vi "Load Variables.vi"(6 "Constants":refnum<class "Sequence Constants.lvclass">, 8 "error in (no error)":refnum<class "MultiErrors.lvclass">, 10 "Config Element":refnum<class "Config Element.lvclass">) -> (0 "error out":refnum<class "MultiErrors.lvclass">, 2 "Variables":map{string, T1}(c390))   [LabVIEW 2020, in "VolatusSeqConfig.lvlib" / "Sequence Config.lvclass"]
uses:
  Sequence Config.lvclass
  VolatusErrorUtilities/MultiErrors/MultiErrors.lvclass
  lv-cdm/CDM-Config/Config Element/Config Element.lvclass
  Variable.ctl
  VolatusErrorUtilities/MultiErrors/MultiErrors.lvclass/MultiErrors.ctl
  Sequence Config.lvclass/Sequence Config.ctl
  VolatusSeqConfig.lvlib
  Sequence Constants/Sequence Constants.lvclass
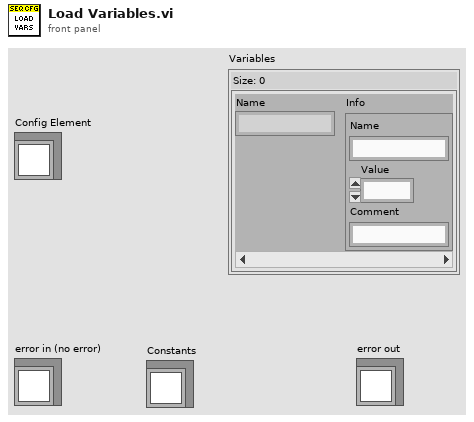
[diagram p1: front panel]
types:
  T1 = typedef "VolatusSeqConfig.lvlib/Variable.ctl" = cluster{"Name":string, "Value":dbl, "Comment":string}
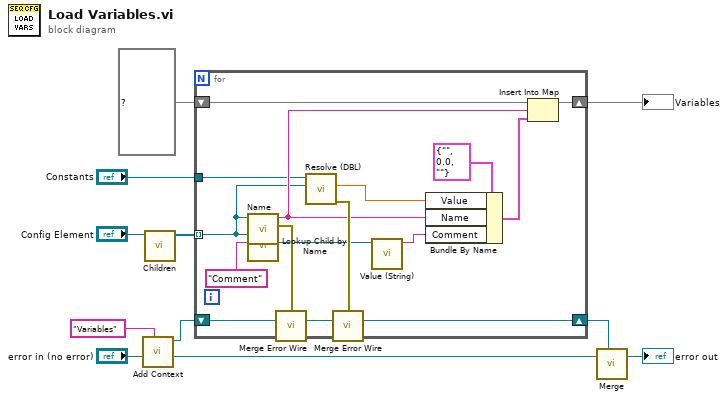
[diagram p0: block diagram]
diagram:
  n1 = call "Add Context.vi"("Context"="Variables", "MultiErrors in"="error in (no error)") -> ("Original Context"=w4:refnum<class "MultiErrors.lvclass">, "Added Context"=w3:refnum<class "MultiErrors.lvclass">)  [unwired: 8 in]
  n2 = call "Children.vi"("Config Element in"="Config Element") -> ("Elements"=w10:refnum<class "Config Element.lvclass">[])  [unwired: 9 in, 1 out]
  n3 = for {
    tunnel: w10 -> [w13] mode=indexing
    shift-right: [w23] -> w8
    shift-left: map{string, T1} {} ("Variables") -> [w24]
    shift-right: [w15] -> w6
    shift-left: w3 -> [w17]
    tunnel: "Constants" -> [w14]
    n4 = call "Name.vi"("Config Element in"=w13) -> ("error out"=w26:errorcluster, "Name"=w21:string)  [unwired: 9 in]
    n5 = call "Lookup Child by Name.vi"("Name"="Comment", "Config Element in"=w13) -> ("Child"=w19:refnum<class "Config Element.lvclass">)  [unwired: 6 in, 3 out]
    n6 = call "Merge Error Wire.vi"("error in (no error)"=w26, "MultiErrors in"=w17) -> ("MultiErrors out"=w16:refnum<class "MultiErrors.lvclass">)  [unwired: 13 in]
    n7 = call "Resolve (DBL).vi"("Element"=w13, "Sequence Constants in"=w14) -> ("error out"=w27:errorcluster, "DBL Value"=w12:dbl)  [unwired: 7 in, 1 out]
    n8 = call "Merge Error Wire.vi"("error in (no error)"=w27, "MultiErrors in"=w16) -> ("MultiErrors out"=w15:refnum<class "MultiErrors.lvclass">)  [unwired: 13 in]
    n9 = call "Value (String).vi"("Config Element in"=w19) -> ("String Value"=w18:string)  [unwired: 9 in, 1 out]
    n10 = Bundle By Name(cluster=T1 {"Name"="", "Value"=0.0, "Comment"=""} ("Variable"), "Value"=w12, "Name"=w21, "Comment"=w18) -> (w22:T1)
    n11 = Insert Into Map(map in=w24, key=w21, value=w22) -> (map out=w23:map{string, T1})  [unwired: 2 out]
  }
  "Variables" <- w8
  n12 = call "Merge.vi"("First Error In"=w4, "Second Error In"=w6) -> ("MultiErrors out"=→"error out":refnum<class "MultiErrors.lvclass">)  [unwired: 5 in]
